vi "save_jv_data.vi"(0 "File path for jv data (without scan direction)":path, 1 "Scan settings":T1 {"Settling delay (s)" min=0.0; "J-t illumination" items=["Light only", "Dark only", "Light then dark", "Dark then light"]; "Measurement speed" items=["Fast", "Normal", "High accuracy"]; "Illumination" items=["Light only", "Dark only", "Light then dark", "Dark then light"]; "Only repeat for best pixel" items=["only for best pixel", "for best 2 pixels", "for best 3 pixels", "for best 4 pixels", "for best 5 pixels", "for best 6 pixels", "for best 7 pixels", "for all pixels"]; "No. of repeat scans" min=1.0 step=1.0; "Max power best pixel only" items=["only the best pixel", "the best 2 pixels", "the best 3 pixels", "the best 4 pixels", "the best 5 pixels", "the best 6 pixels", "the best 7 pixels", "all pixels"]; "J-t best pixel only" items=["only the best pixel", "the best 2 pixels", "the best 3 pixels", "the best 4 pixels", "the best 5 pixels", "the best 6 pixels", "the best 7 pixels", "all pixels"]; "J-t measurement speed" items=["Fast", "Normal", "High Accuracy"]; "Stabilisation mode" items=["V", "I"]; "Measurement delay (ms)" min=10.0}, 2 "Cell details cluster":T2={"Cell Position"=16, "Cell Label"="", "Pixel to measure"=0, "Area (cm^2)"=0.126, "Variable"="", "Variable value"="", "Scan settings in queue"=0, "Light or dark"="", "Measurement type"=""} {"Pixel to measure" items=["All", "1", "2", "3", "4", "5", "6", "7", "8"]}, 7 "Scan direction":i32, 9 "Data Array":dbl[][](array[numeric]), 12 "intensity (no. of suns)":string) -> (4 "File path for JV data (without direction)":path, 6 "File path for JV image":path, 8 "j-v metrics":string[](array[string]), 10 "File path out (with scan direction)":string, 15 "scan direction":string)   [LabVIEW 2016]
uses:
  TypeDefs/scan_settings.ctl
  <vilib>/Utility/file.llb/Write Delimited Spreadsheet (string).vi
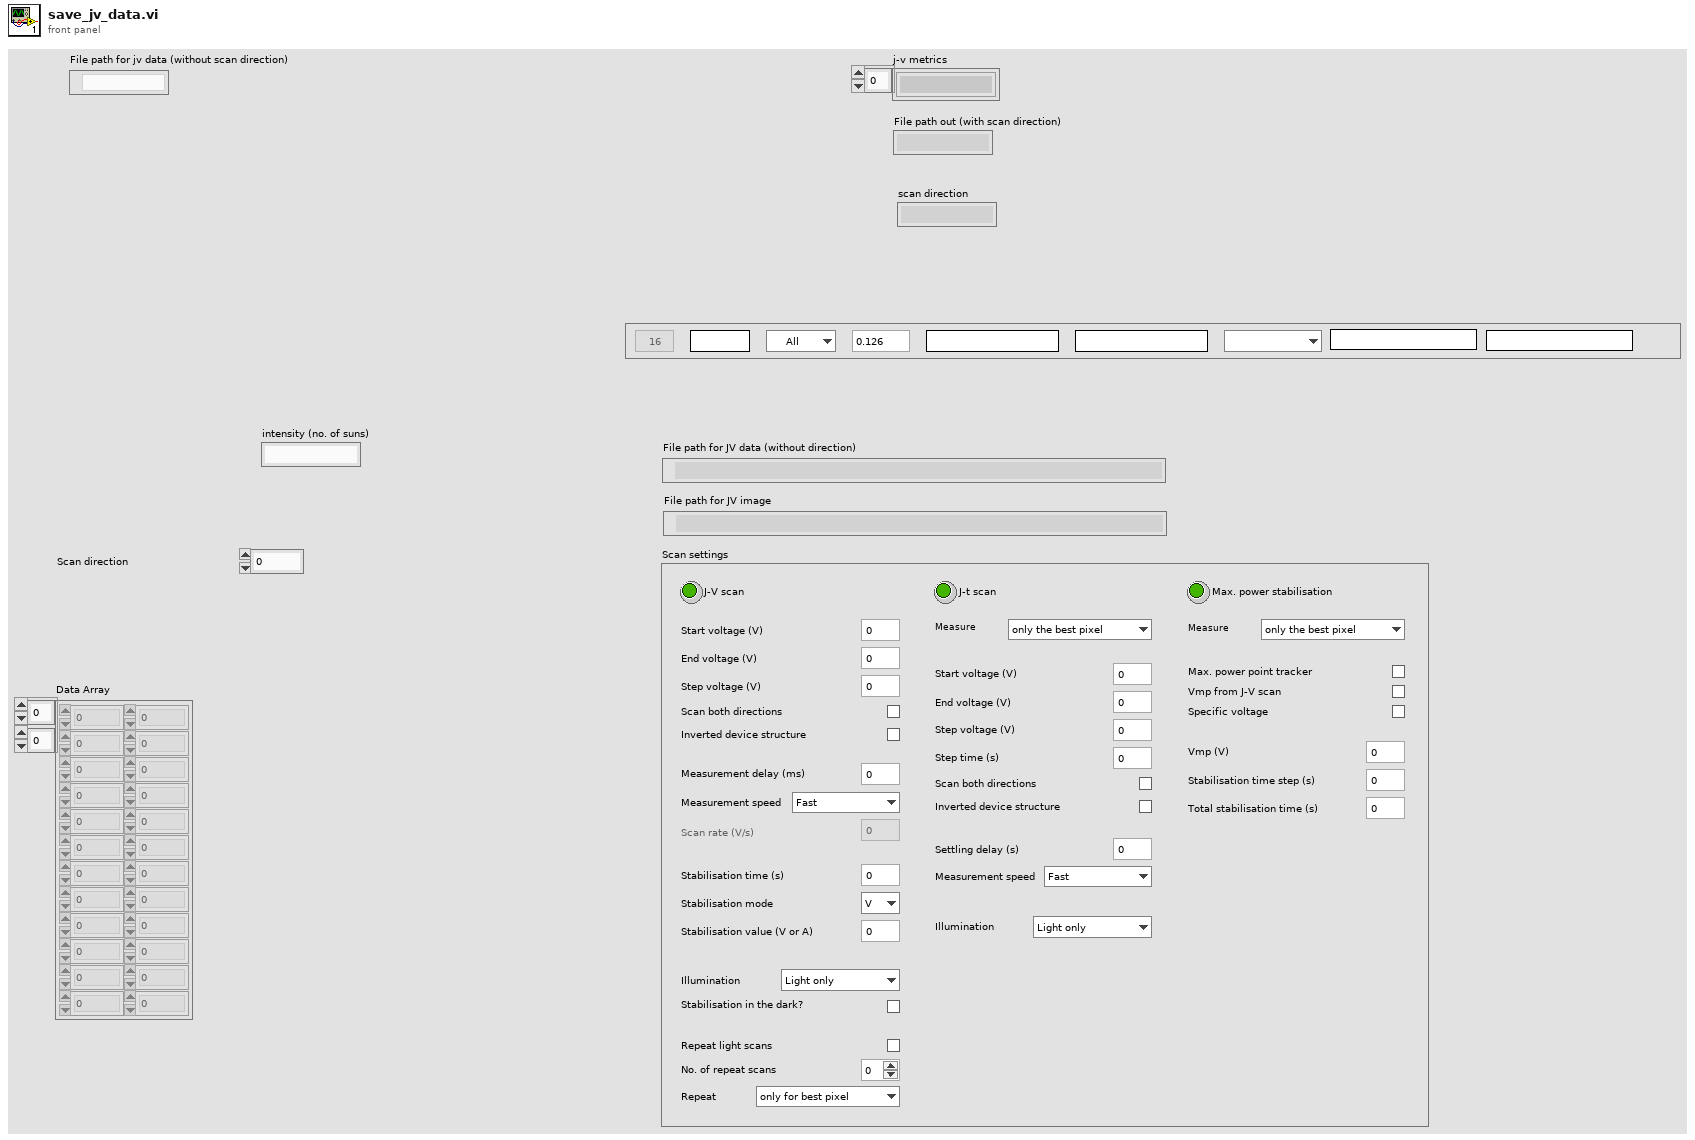
[diagram p1: front panel]
types:
  T1 = typedef "scan_settings.ctl" = cluster{"J-V scan":bool, "Start voltage (V)":dbl, "End voltage (V)":dbl, "Step voltage (V)":dbl, "Scan both directions":bool, "Inverted device structure":bool, "Measurement delay (ms)":dbl, "Measurement speed":u8, "Scan rate (V/s)":dbl, "Stabilisation time (s)":dbl, "Stabilisation mode":u16, "Stabilisation value (V or A) ":dbl, "Illumination":u16, "Stabilisation in the dark?":bool, "Repeat light scans":bool, "No. of repeat scans":dbl, "Only repeat for best pixel":u16, "J-t scan":bool, "J-t best pixel only":u16, "J-t start voltage (V)":dbl, "J-t end voltage (V)":dbl, "J-t step voltage (V)":dbl, "Step time (s)":dbl, "J-t scan both directions":bool, "J-t inverted device structure":bool, "Settling delay (s)":dbl, "J-t measurement speed":u16, "J-t illumination":u16, "Max. power stabilisation":bool, "Max power best pixel only":u16, "Max. power point tracker":bool, "Vmp from J-V scan":bool, "Max P stab. Specific voltage":bool, "Vmp (V)":dbl, "Stabilisation time step (s)":dbl, "Total stabilisation time (s)":dbl}
  T2 = cluster{"Cell Position":i32, "Cell Label":string, "Pixel to measure":u16, "Area (cm^2)":dbl, "Variable":string, "Variable value":string, "Scan settings in queue":u16, "Light or dark":string, "Measurement type":string}
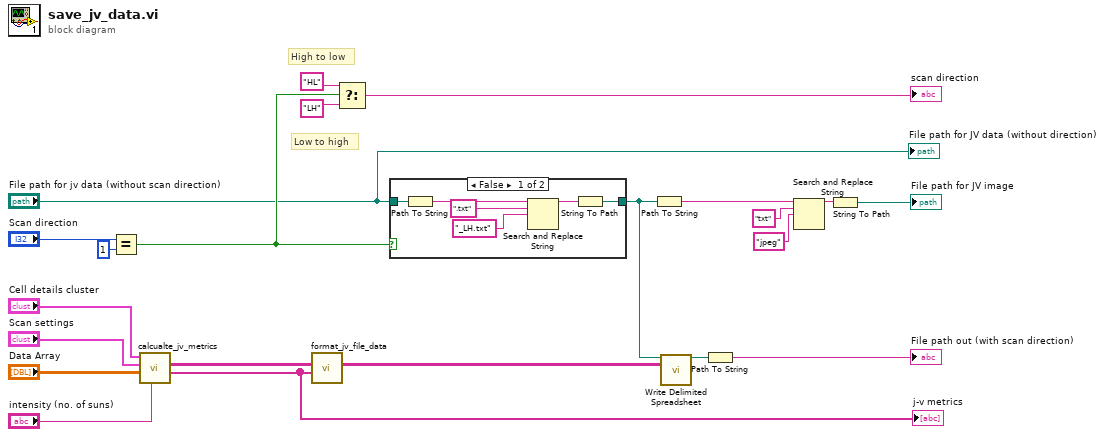
[diagram p0: block diagram]
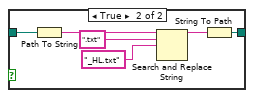
[diagram p2: hidden frame]
diagram:
  # "Low to high"
  # "High to low"
  n1 = Equal?(x="Scan direction", y=1) -> (x = y?=w11:bool)
  n2 = call "calcualte_jv_metrics.vi"("intensity (no. of suns)"="intensity (no. of suns)", "Data Array"="Data Array", "Scan settings"="Scan settings", "Cell details cluster"="Cell details cluster") -> ("j-v metrics"=w2:string[], "j-v data"=w3:string[][])  [unwired: 6 in]
  "j-v metrics" <- w2
  n3 = call "format_jv_file_data.vi"("j-v metrics"=w2, "j-v data"=w3) -> ("file data"=w4:string[][])  [unwired: 9 in]
  n4 = Select(t="HL", s=w11, f="LH") -> (s? t:f=→"scan direction":string)
  n5 = case shown="False" w11 {
    tunnel: "File path for jv data (without scan direction)" -> [w23 w30]
    tunnel: [w24 w29] -> w12
    frame False {
      n6 = Path To String(path=w23) -> (string=w27:string)
      n7 = Search and Replace String(input string=w27, search string=".txt", replace string="_LH.txt" ("replace string (\"\")")) -> (result string=w28:string)  [unwired: 5 in, 3 out]
      n8 = String To Path(string=w28) -> (path=w24:path)
    }
    frame True {
      n9 = Path To String(path=w30) -> (string=w33:string)
      n10 = Search and Replace String(input string=w33, search string=".txt", replace string="_HL.txt" ("replace string (\"\")")) -> (result string=w34:string)  [unwired: 5 in, 3 out]
      n11 = String To Path(string=w34) -> (path=w29:path)
    }
  }
  n12 = Path To String(path=w12) -> (string=w13:string)
  n13 = call-poly <vilib>:"Write Delimited Spreadsheet.vi"("file path (dialog if empty)"=w12, "2D data"=w4) -> ("new file path (Not A Path if cancelled)"=w14:path)  [unwired: 12 in, 1 out]
  n14 = Path To String(path=w14) -> (string=→"File path out (with scan direction)":string)
  n15 = Search and Replace String(input string=w13, search string="txt", replace string="jpeg") -> (result string=w20:string)  [unwired: 5 in, 3 out]
  n16 = String To Path(string=w20) -> (path=→"File path for JV image":path)
  "File path for JV data (without direction)" <- "File path for jv data (without scan direction)"
